vi "ep_dB Convert.vi"(4 "demodulated? (F)":bool, 6 "dB on? (T)":bool=TRUE, 8 "phase output? (F)":bool, 11 "spectrum in":cdb[](array[numeric])) -> (0 "phase":dbl[](array[numeric]), 3 "magnitude":dbl[](array[numeric]))   [LabVIEW 2014, in "NI_EP_Motor Monitoring.lvlib"]
uses:
  <vilib>/addons/Electrical Power/Motor Monitoring/NI_EP_Motor Monitoring.lvlib
  <vilib>/Analysis/NI_AALPro.lvlib
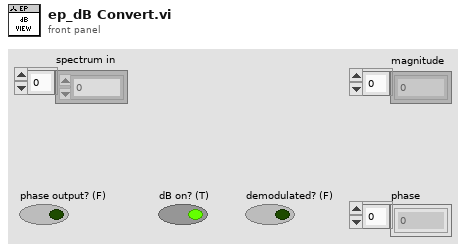
[diagram p1: front panel]
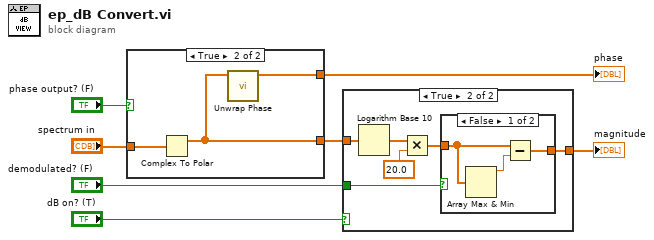
[diagram p0: block diagram]
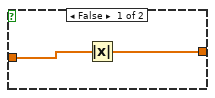
[diagram p2: hidden frame]
diagram:
  n1 = case shown="True" "phase output? (F)" {
    tunnel: "spectrum in" -> [w9 w12]
    tunnel: [w8 w11] -> w2
    tunnel: [_ w10] -> w1
    frame False {
      n2 = Absolute Value(x=w9) -> (abs(x)=w8:dbl[])
    }
    frame True {
      n3 = Complex To Polar(r * e^(i*theta)=w12) -> (r=w11:dbl[])  [unwired: 1 out]
      n4 = call <vilib>:"Unwrap Phase.vi"("Phase"=w11) -> ("Unwrapped Phase"=w10:dbl[])  [unwired: 9 in, 1 out]
    }
  }
  "phase" <- w1
  n5 = case shown="True" "dB on? (T)" {
    tunnel: w2 -> [w13 w14]
    tunnel: "demodulated? (F)" -> [_ w16]
    tunnel: [w13 w15] -> w6
    frame False {
    }
    frame True {
      n6 = Logarithm Base 10(1:w14) -> (0:w19:dbl[])
      n7 = Multiply(x=w19, y=20.0) -> (x*y=w17:dbl[])
      n8 = case shown="False" w16 {
        tunnel: w17 -> [w21 w23]
        tunnel: [w22 w23] -> w15
        frame False {
          n9 = Array Max & Min(array=w21) -> (max value=w20:dbl)  [unwired: 3 out]
          n10 = Subtract(x=w21, y=w20) -> (x-y=w22:dbl[])
        }
        frame True {
        }
      }
    }
  }
  "magnitude" <- w6
